vi "Select ctrls and indicators visibility.vi"(8 "error in (no error)":errorcluster, 10 "Combo Box":string(combo), 11 "cluster ref":refnum<vi>) -> (0 "error out":errorcluster)   [LabVIEW 2015]
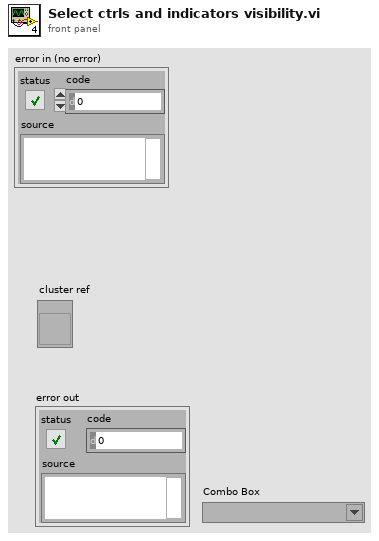
[diagram p1: front panel]
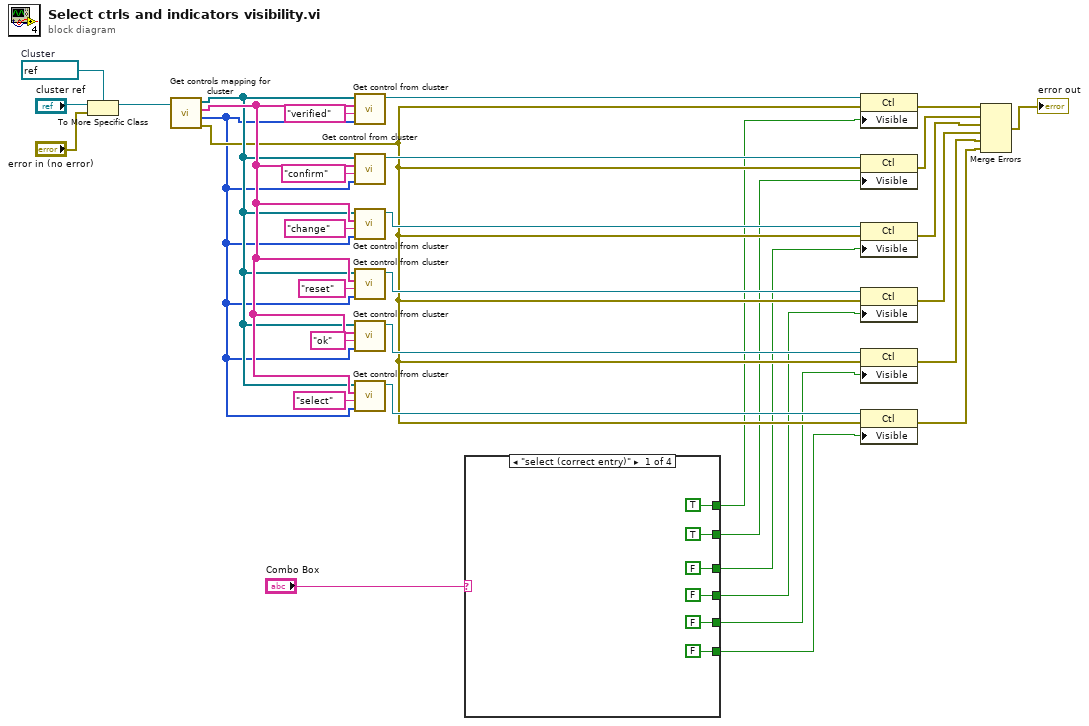
[diagram p0: block diagram]
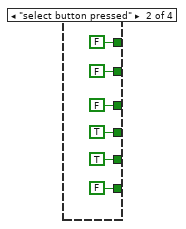
[diagram p2: hidden frame]
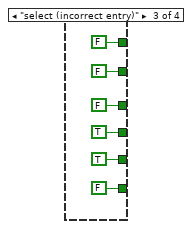
[diagram p3: hidden frame]
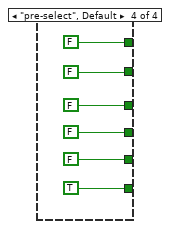
[diagram p4: hidden frame]
diagram:
  w10 = refnum<vi> refnum  # Cluster
  n1 = To More Specific Class(target class=w10, reference="cluster ref", error in="error in (no error)") -> (specific class reference=w11:refnum<vi>)  [unwired: 1 out]
  n2 = call "Get controls mapping for cluster.vi"("Ctl Refnum"=w11) -> ("error out"=w21:errorcluster, "Mapping array"=w9:i32[], "Boolean labels array"=w28:string[], "Controls[]"=w27:refnum<vi>[])  [unwired: 7 in]
  n3 = call "Get control from cluster.vi"("Mapping array"=w9, "Combo Box"="verified", "Array of booleans"=w28, "Controls[]"=w27) -> ("control ref"=w33:refnum<vi>)  [unwired: 7 in]
  n4 = call "Get control from cluster.vi"("Mapping array"=w9, "Combo Box"="confirm", "Array of booleans"=w28, "Controls[]"=w27) -> ("control ref"=w26:refnum<vi>)  [unwired: 7 in]
  n5 = call "Get control from cluster.vi"("Mapping array"=w9, "Combo Box"="change", "Array of booleans"=w28, "Controls[]"=w27) -> ("control ref"=w25:refnum<vi>)  [unwired: 7 in]
  n6 = call "Get control from cluster.vi"("Mapping array"=w9, "Combo Box"="reset", "Array of booleans"=w28, "Controls[]"=w27) -> ("control ref"=w24:refnum<vi>)  [unwired: 7 in]
  n7 = call "Get control from cluster.vi"("Mapping array"=w9, "Combo Box"="ok", "Array of booleans"=w28, "Controls[]"=w27) -> ("control ref"=w23:refnum<vi>)  [unwired: 7 in]
  n8 = call "Get control from cluster.vi"("Mapping array"=w9, "Combo Box"="select", "Array of booleans"=w28, "Controls[]"=w27) -> ("control ref"=w22:refnum<vi>)  [unwired: 7 in]
  n9 = case shown="\"select (correct entry)\"" "Combo Box" {
    tunnel: [TRUE FALSE FALSE FALSE] -> w19
    tunnel: [TRUE FALSE FALSE FALSE] -> w18
    tunnel: [FALSE FALSE FALSE FALSE] -> w17
    tunnel: [FALSE TRUE TRUE FALSE] -> w16
    tunnel: [FALSE TRUE TRUE FALSE] -> w15
    tunnel: [FALSE FALSE FALSE TRUE] -> w14
    frame "select (correct entry)" {
    }
    frame "select button pressed" {
    }
    frame "select (incorrect entry)" {
    }
    frame "pre-select", Default {
    }
  }
  n10 = property class="Ctl"(reference=w33, error in=w21, "Visible"=w19) -> (error out=w6:errorcluster)  [unwired: 1 out]
  n11 = property class="Ctl"(reference=w26, error in=w21, "Visible"=w18) -> (error out=w7:errorcluster)  [unwired: 1 out]
  n12 = property class="Ctl"(reference=w25, error in=w21, "Visible"=w17) -> (error out=w5:errorcluster)  [unwired: 1 out]
  n13 = property class="Ctl"(reference=w24, error in=w21, "Visible"=w16) -> (error out=w4:errorcluster)  [unwired: 1 out]
  n14 = property class="Ctl"(reference=w23, error in=w21, "Visible"=w15) -> (error out=w3:errorcluster)  [unwired: 1 out]
  n15 = property class="Ctl"(reference=w22, error in=w21, "Visible"=w14) -> (error out=w2:errorcluster)  [unwired: 1 out]
  n16 = Merge Errors(w6, w7, w5, w4, w3, w2) -> (→"error out":errorcluster)
